vi "SetOpMode.vi"(8 "error in (no error)":errorcluster, 10 "Op Mode":u8, 11 "BME680 in":refnum<class "BME680.lvclass">) -> (0 "error out":errorcluster, 3 "BME680 out":refnum<class "BME680.lvclass">)   [LabVIEW 2022 SP3, in "BME680.lvlib" / "BME680.lvclass"]
uses:
  BME680.lvclass
  BME680.lvclass/BME680.ctl
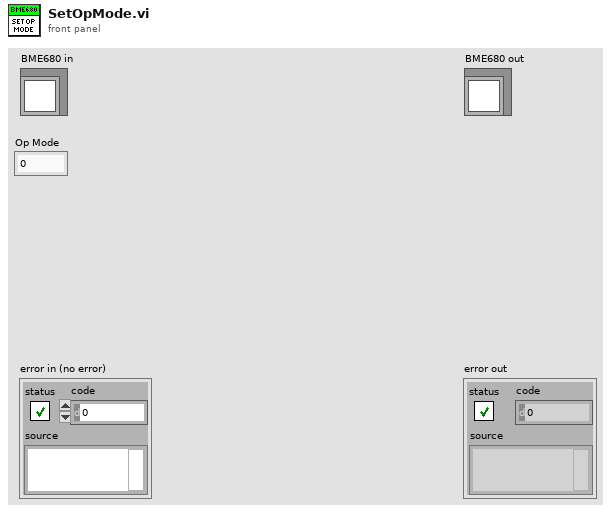
[diagram p1: front panel]
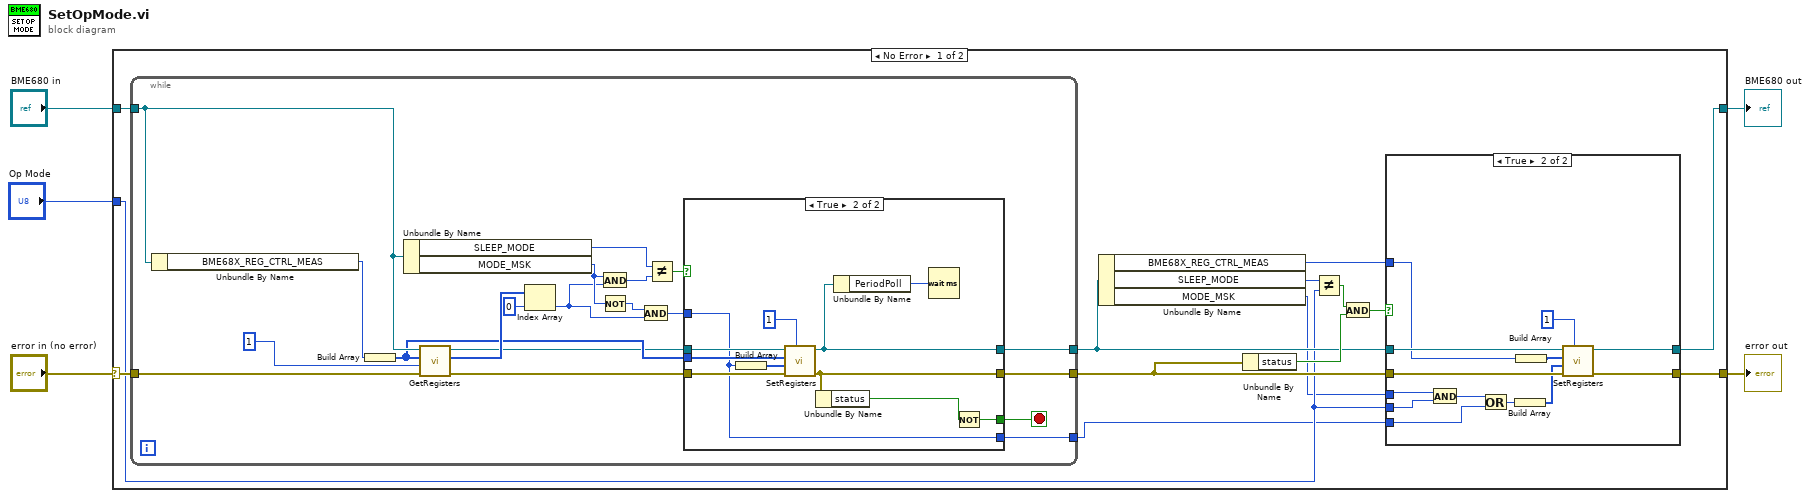
[diagram p0: block diagram]
diagram:
  n1 = case shown="No Error" "error in (no error)" {
    selector: "error in (no error)" -> [w19 w69]
    tunnel: [w9 w69] -> w4
    tunnel: [w8 w68] -> w2
    tunnel: "BME680 in" -> [w18 w68]
    tunnel: "Op Mode" -> [w12 _]
    frame No Error {
      n2 = while {
        tunnel: w19 -> [w54]
        tunnel: w18 -> [w49]
        tunnel: [w37] -> w13
        tunnel: [w36] -> w17
        tunnel: [w35] -> w6
        stop <- w42 stop-if-true
        n3 = Unbundle By Name(w49) -> ("BME68X_REG_CTRL_MEAS"=w53:u8)
        n4 = Build Array(w53) -> (w45:u8[])
        n5 = Unbundle By Name(w49) -> ("SLEEP_MODE"=w48:u8, "MODE_MSK"=w41:u8)
        n6 = call-dynamic "GetRegisters.vi"("error in (no error)"=w54, "Lenght"=u8 1, "Addr"=w45, "BME680 in"=w49) -> ("error out"=w46:errorcluster, "Data out"=w51:u8[], "BME680 out"=w43:refnum<class "BME680.lvclass">)  [unwired: 5 in]
        n7 = Index Array(array=w51, index=0) -> (element=w39:u8)
        n8 = And(x=w41, y=w39) -> (x .and. y?=w44:u8)
        n9 = Not(x=w41) -> (.not. x?=w40:u8)
        n10 = And(x=w40, y=w39) -> (x .and. y?=w38:u8)
        n11 = Not Equal?(x=w48, y=w44) -> (x != y?=w47:bool)
        n12 = case shown="True" w47 {
          tunnel: w46 -> [w55 w67]
          tunnel: w45 -> [_ w66]
          tunnel: w43 -> [w56 w64]
          tunnel: [w55 w63] -> w36
          tunnel: [_ w61] -> w42
          tunnel: [w56 w60] -> w37
          tunnel: w38 -> [_ w57]
          tunnel: [_ w57] -> w35
          frame False {
          }
          frame True {
            n13 = Build Array(w57) -> (w58:u8[])
            n14 = call-dynamic "SetRegisters.vi"("Lenght"=1, "error in (no error)"=w67, "Register Data"=w58, "Register Addres"=w66, "BME680 in"=w64) -> ("error out"=w63:errorcluster, "BME680 out"=w60:refnum<class "BME680.lvclass">)  [unwired: 5 in]
            n15 = Unbundle By Name(w63) -> ("status"=w62:bool)
            n16 = Unbundle By Name(w60) -> ("PeriodPoll"=w59:i32)
            n17 = Wait (ms)(milliseconds to wait=w59) -> ()  [unwired: 1 out]
            n18 = Not(x=w62) -> (.not. x?=w61:bool)
          }
        }
      }
      n19 = Unbundle By Name(w13) -> ("BME68X_REG_CTRL_MEAS"=w10:u8, "SLEEP_MODE"=w11:u8, "MODE_MSK"=w7:u8)
      n20 = Unbundle By Name(w17) -> ("status"=w16:bool)
      n21 = Not Equal?(x=w11, y=w12) -> (x != y?=w15:bool)
      n22 = And(x=w15, y=w16) -> (x .and. y?=w14:bool)
      n23 = case shown="True" w14 {
        tunnel: w12 -> [_ w27]
        tunnel: w17 -> [w20 w34]
        tunnel: w13 -> [w21 w33]
        tunnel: w10 -> [_ w32]
        tunnel: [w20 w30] -> w9
        tunnel: [w21 w29] -> w8
        tunnel: w7 -> [_ w26]
        tunnel: w6 -> [_ w24]
        frame False {
        }
        frame True {
          n24 = And(x=w26, y=w27) -> (x .and. y?=w25:u8)
          n25 = Or(x=w25, y=w24) -> (x .or. y?=w23:u8)
          n26 = Build Array(w23) -> (w22:u8[])
          n27 = Build Array(w32) -> (w31:u8[])
          n28 = call-dynamic "SetRegisters.vi"("Lenght"=1, "error in (no error)"=w34, "Register Data"=w22, "Register Addres"=w31, "BME680 in"=w33) -> ("error out"=w30:errorcluster, "BME680 out"=w29:refnum<class "BME680.lvclass">)  [unwired: 5 in]
        }
      }
    }
    frame Error {
    }
  }
  "error out" <- w4
  "BME680 out" <- w2
